vi "Save File.vi"(0 "Save Options":T1={"Component Name"="", "Image Type"=enum."PNG", "Save As"=enum."Save", "Image"=refnum, "PostProcessed?"=FALSE, "Color Palette"=[], "Display Range"={"Maximum"=0, "Minimum"=0}, "Image Refnum"=refnum, "save name"=FALSE, "Dynamic Filter"=FALSE}, 11 "Error in (no error)":errorcluster, 13 "Save Location":enum16{"Primary", "Secondary"}(ring)) -> (4 "Last Saved File Name":string, 8 "Last Saved File Path":path, 15 "Error out":errorcluster)   [LabVIEW 2021]
uses:
  Controls/Save VI States.ctl
  <vilib>/vision/Image Controls.llb/IMAQ Image.ctl
  Controls/Image Type.ctl
  Controls/Save Options.ctl
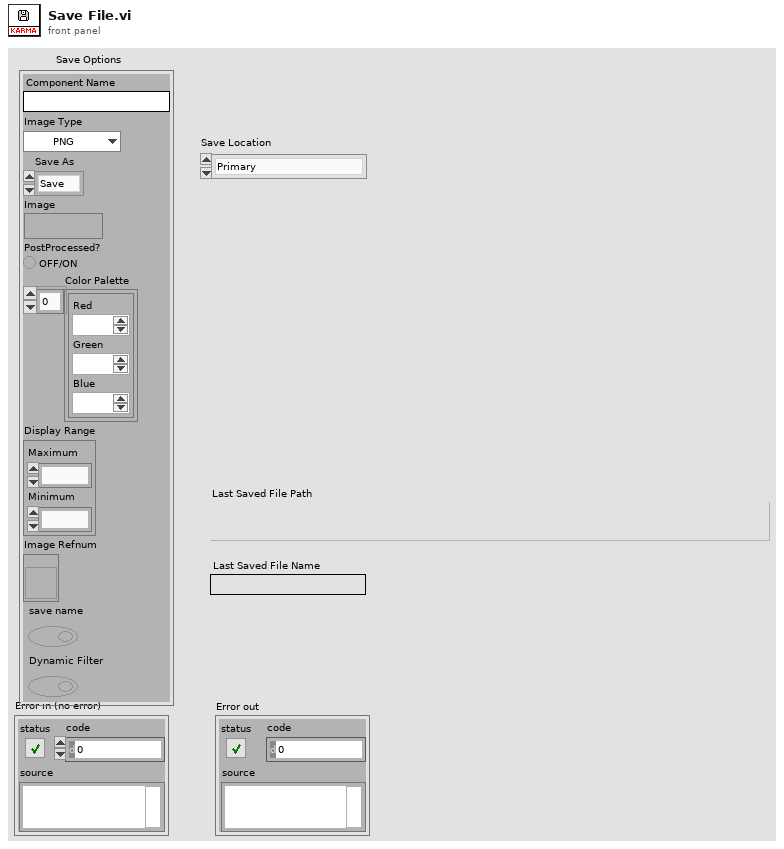
[diagram p1: front panel]
types:
  T1 = typedef "Save Options.ctl" = cluster{"Component Name":string, "Image Type":T2, "Save As":enum16{"Save", "SaveAsOK", "SaveAsNOTOK"}, "Image":T3, "PostProcessed?":bool, "Color Palette":cluster{"Red":u8, "Green":u8, "Blue":u8}[], "Display Range":cluster{"Maximum":i32, "Minimum":i32}, "Image Refnum":refnum<vi>, "save name":bool, "Dynamic Filter":bool}
  T2 = typedef "Image Type.ctl" = enum16{"JPEG", "BMP", "PNG", "TIFF", "DICOM", "RAW"}
  T3 = typedef "IMAQ Image.ctl" = refnum<image>
  T4 = typedef "Save VI States.ctl" = enum16{"Initialize", "Check File Paths", "Target Folder Selection", "Check File Count", "Save File", "Exit"}
  T5 = enum16{"Init Counter", "Read Last Value", "Write Last Value", "Reset Counter", "Increment by 1", "Decrement by 1", "Get Current Count"}
  T6 = cluster{"Last Saved Path":path, "Component name":string}
  T7 = typedef "Application Settings.ctl" = cluster{"Sensor Settings":cluster{"Sensor Type Selection":enum32{"IDS Sensor", "Select Sensor"}, "Select Sensor":T8, "Sensor ID":u32, "Bit Depth":enum16{"<Select>", "8 bits", "16 bits"}}, "Save Options":cluster{"Primary Storage Location":path, "Backup Storage Location":path, "Enable Primary":bool, "Enable Secondary":bool}, "Other Settings":cluster{"Show Image Averaging Option":bool}}
  T8 = typedef "IMAQdx.ctl" = refnum<k21>
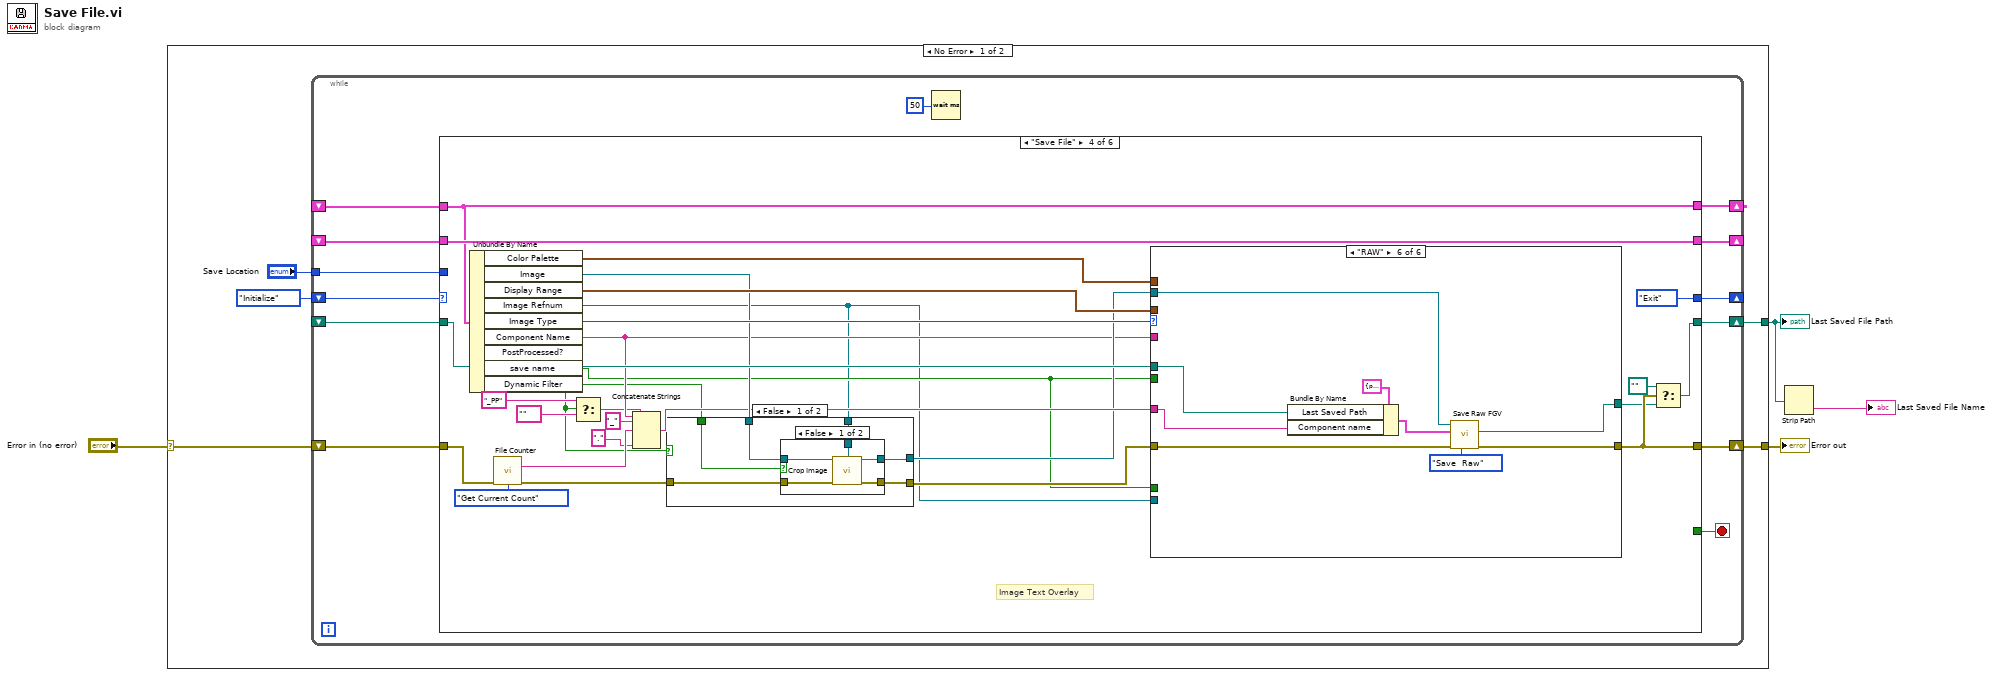
[diagram p0: block diagram]
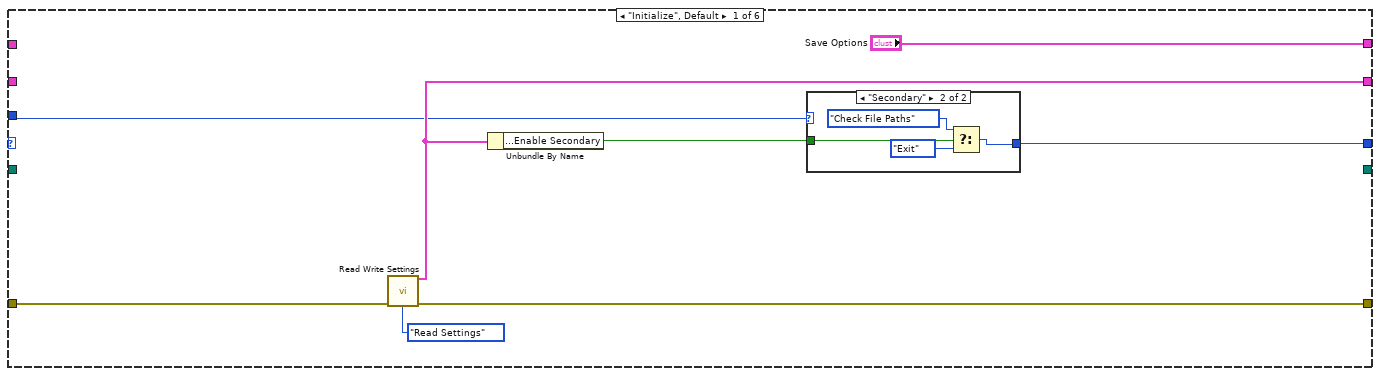
[diagram p2: hidden frame]
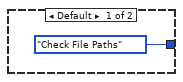
[diagram p3: hidden frame]
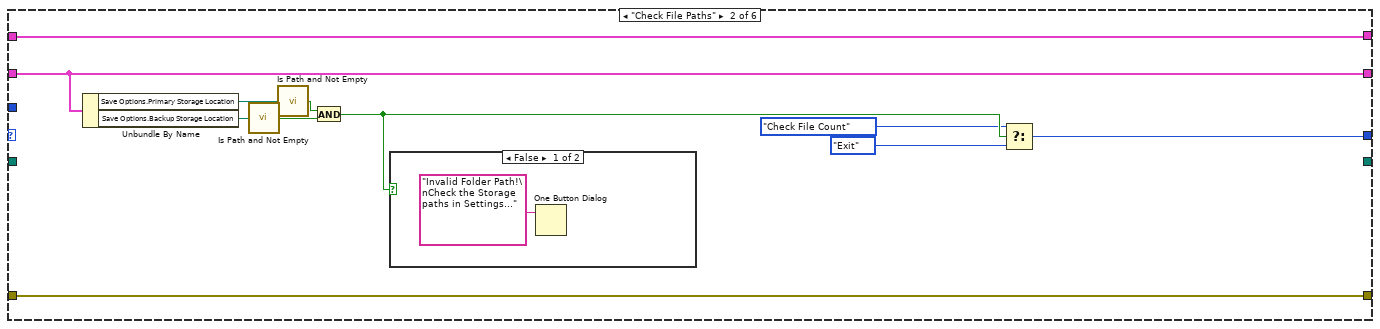
[diagram p4: hidden frame]
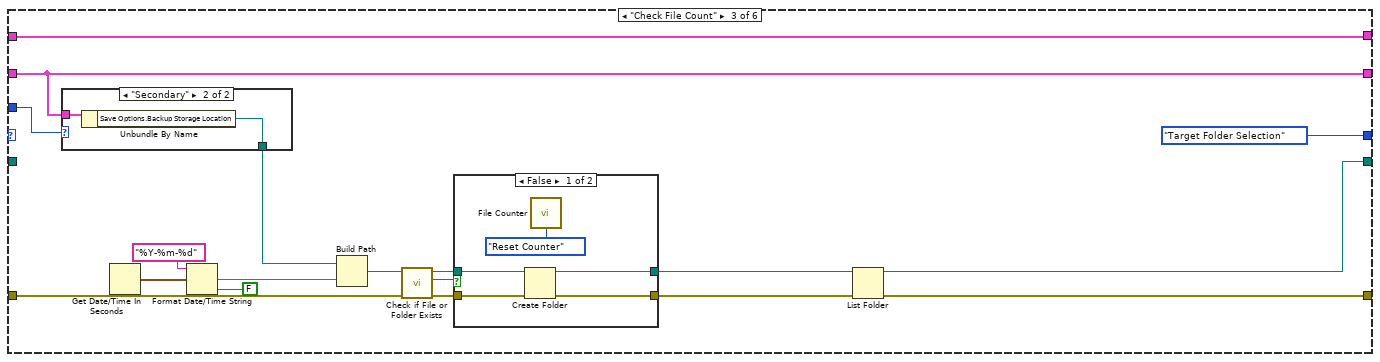
[diagram p6: hidden frame]
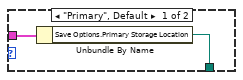
[diagram p7: hidden frame]
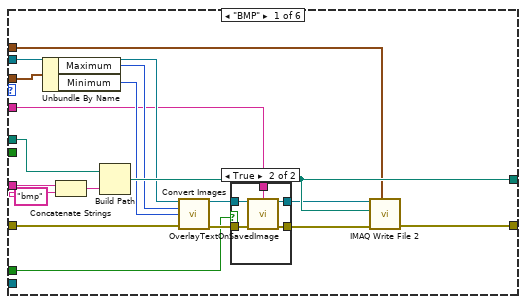
[diagram p11: hidden frame]
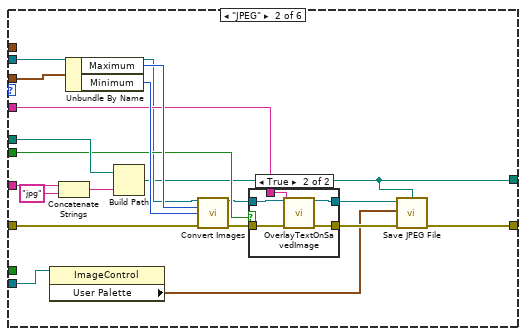
[diagram p13: hidden frame]
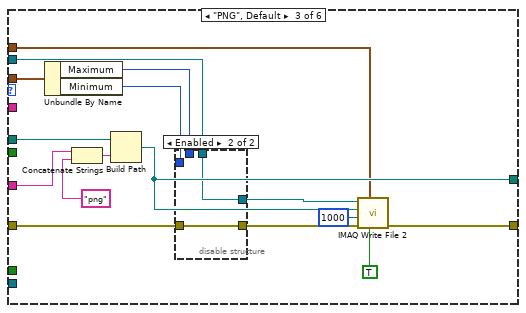
[diagram p15: hidden frame]
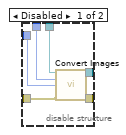
[diagram p16: hidden frame]
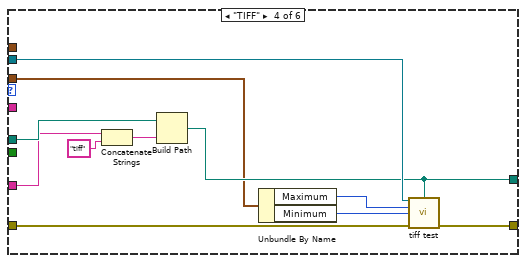
[diagram p17: hidden frame]
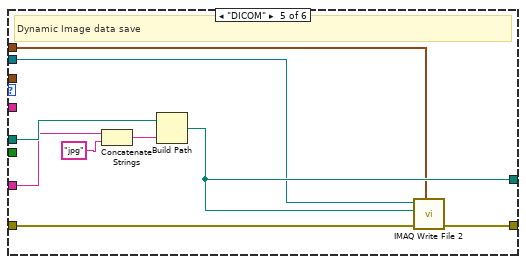
[diagram p18: hidden frame]
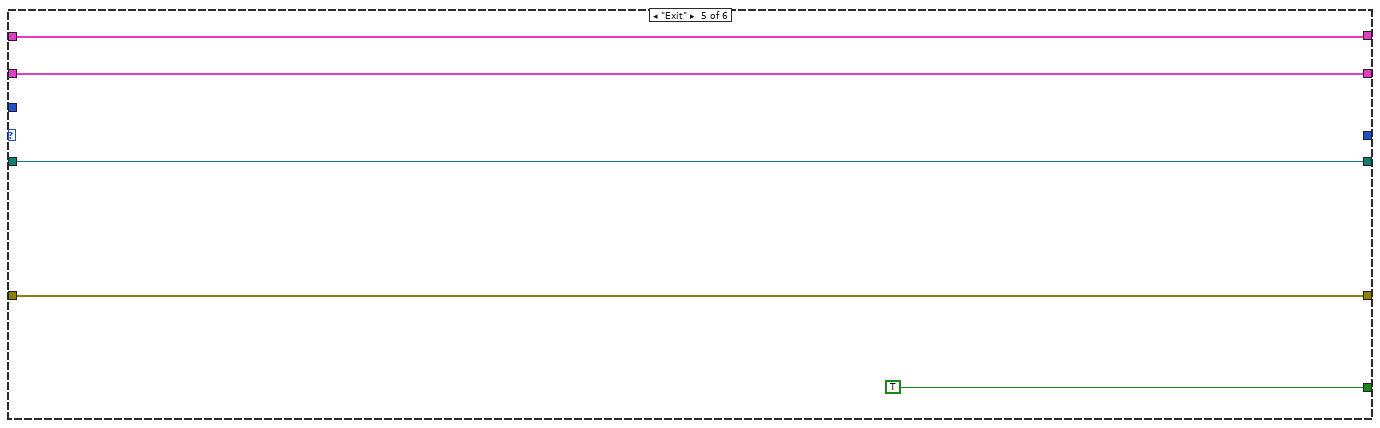
[diagram p19: hidden frame]
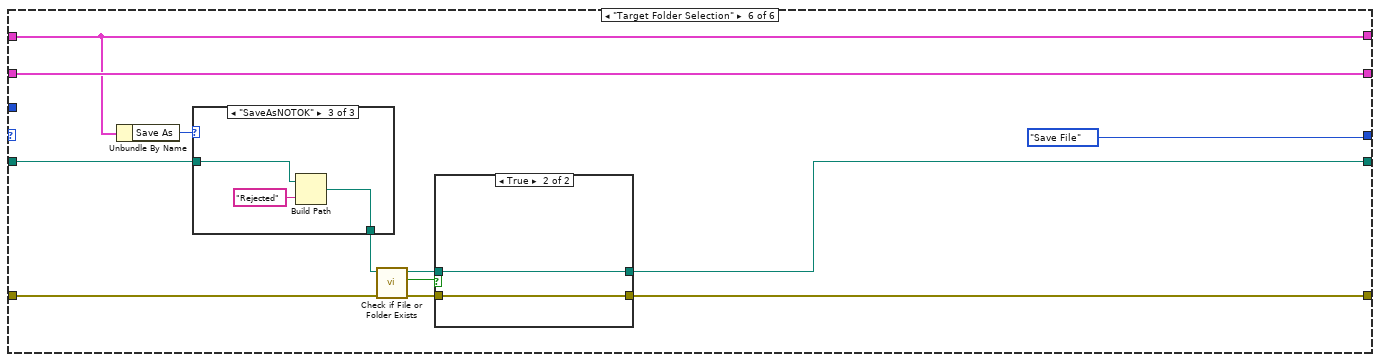
[diagram p20: hidden frame]
diagram:
  n1 = case shown="No Error" "Error in (no error)" {
    selector: "Error in (no error)" -> [w5 w255]
    tunnel: [w7 _] -> w2
    tunnel: [w6 w255] -> w4
    frame No Error {
      n2 = while {
        shift-right: [w14] -> _
        shift-left: Save_VI_States."Initialize" -> [w22]
        shift-right: [w20] -> _
        shift-left: _ -> [w19]
        shift-right: [w16] -> _
        shift-left: _ -> [w15]
        shift-right: [w13] -> w7
        shift-left: _ -> [w12]
        tunnel: "Save Location" -> [w11]
        shift-right: [w17] -> w6
        shift-left: w5 -> [w18]
        stop <- w21 stop-if-true
        n3 = case shown="\"Save File\"" w22 {
          tunnel: [_ _ _ _ TRUE _] -> w21
          tunnel: ["Save Options" w46 w65 w102 w228 w240] -> w20
          tunnel: w19 -> [_ w46 w65 w102 w228 w240]
          tunnel: w18 -> [w28 w38 w53 w89 w226 w233]
          tunnel: [w27 w38 w52 w97 w226 w232] -> w17
          tunnel: [w26 w41 w51 w105 w227 w241] -> w16
          tunnel: w15 -> [_ w41 w51 w105 w227 w241]
          tunnel: [w23 w39 Save_VI_States."Target Folder Selection" Save_VI_States."Exit" _ Save_VI_States."Save File"] -> w14
          tunnel: [_ _ w50 w94 w225 w231] -> w13
          tunnel: w12 -> [_ _ _ w98 w225 w234]
          tunnel: w11 -> [w25 _ w48 _ _ _]
          frame "Initialize", Default {
            n4 = call "Read Write Settings.vi"("error in (no error)"=w28, "Operations"=enum16{"Read Settings", "Write Settings"}."Read Settings") -> ("Settings Out"=w26:T7, "error out"=w27:errorcluster)  [unwired: 12 in]
            n5 = Unbundle By Name(w26) -> ("Save Options.Enable Secondary"=w24:bool)
            n6 = case shown="\"Secondary\"" w25 {
              tunnel: w24 -> [_ w35]
              tunnel: [Save_VI_States."Check File Paths" w33] -> w23
              frame Default {
              }
              frame "Secondary" {
                n7 = Select(t=Save_VI_States."Check File Paths", s=w35, f=Save_VI_States."Exit") -> (s? t:f=w33:T4)
              }
            }
          }
          frame "Check File Paths" {
            n8 = Unbundle By Name(w41) -> ("Save Options.Primary Storage Location"=w43:path, "Save Options.Backup Storage Location"=w42:path)
            n9 = call <vilib>:"Is Path and Not Empty.vi"("path"=w42) -> ("Is Path and Not Empty?"=w45:bool)  [unwired: 4 in]
            n10 = call <vilib>:"Is Path and Not Empty.vi"("path"=w43) -> ("Is Path and Not Empty?"=w44:bool)  [unwired: 4 in]
            n11 = And(x=w44, y=w45) -> (x .and. y?=w40:bool)
            n12 = case shown="False" w40 {
              frame False {
                n13 = One Button Dialog(message="Invalid Folder Path!\nCheck the Storage paths in Settings...") -> ()  [unwired: 1 in, 1 out]
              }
              frame True {
              }
            }
            n14 = Select(t=Save_VI_States."Check File Count", s=w40, f=Save_VI_States."Exit") -> (s? t:f=w39:T4)
          }
          frame "Check File Count" {
            n15 = case shown="\"Secondary\"" w48 {
              tunnel: [w67 w68] -> w54
              tunnel: w51 -> [w66 w69]
              frame "Primary", Default {
                n16 = Unbundle By Name(w66) -> ("Save Options.Primary Storage Location"=w67:path)
              }
              frame "Secondary" {
                n17 = Unbundle By Name(w69) -> ("Save Options.Backup Storage Location"=w68:path)
              }
            }
            n18 = Get Date/Time In Seconds() -> (seconds since 1Jan1904=w58:timestamp)
            n19 = Format Date/Time String(time format string (%c)="%Y-%m-%d", seconds (now)=w58, UTC format=FALSE) -> (date/time string=w55:string)
            n20 = Build Path(base path=w54, name or relative path=w55) -> (appended path=w64:path)
            n21 = call <vilib>:"Check if File or Folder Exists.vi"("error in (no error)"=w53, "path"=w64) -> ("error out"=w62:errorcluster, "file or folder exists?"=w63:bool, "dup path"=w61:path)  [unwired: 7 in]
            n22 = case shown="False" w63 {
              tunnel: w62 -> [w74 w76]
              tunnel: w61 -> [w72 w75]
              tunnel: [w73 w76] -> w60
              tunnel: [w71 w75] -> w59
              frame False {
                n23 = Create Folder(path (use dialog)=w72, error in=w74) -> (created path=w71:path, error out=w73:errorcluster)  [unwired: 1 in, 1 out]
                n24 = call "File Counter.vi"("Operations"=T5."Reset Counter") -> ()  [unwired: 12 in, 3 out]
              }
              frame True {
              }
            }
            n25 = List Folder(path=w59, error in=w60) -> (path out=w50:path, error out=w52:errorcluster)  [unwired: 2 in, 2 out]
          }
          frame "Save File" {
            # "Image Text Overlay"
            n26 = Unbundle By Name(w102) -> ("Color Palette"=w90:cluster{"Red":u8, "Green":u8, "Blue":u8}[], "Image"=w86:T3, "Display Range"=w91:cluster{"Maximum":i32, "Minimum":i32}, "Image Refnum"=w80:refnum<vi>, "Image Type"=w99:T2, "Component Name"=w82:string, "PostProcessed?"=w87:bool, "save name"=w81:bool, "Dynamic Filter"=w79:bool)
            n27 = call "File Counter.vi"("Error in"=w89, "Operations"=T5."Get Current Count") -> ("Count"=w100:string, "Error out"=w88:errorcluster)  [unwired: 11 in, 1 out]
            n28 = Select(t="_PP" ("string"), s=w87, f="") -> (s? t:f=w77:string)
            n29 = Concatenate Strings(w82, "_" ("f"), w100, w77, "." ("string")) -> (w85:string)
            n30 = case shown="False" w87 {
              tunnel: [w110 w119] -> w84
              tunnel: w86 -> [w109 w120]
              tunnel: [w108 w120] -> w83
              tunnel: w88 -> [w111 w119]
              tunnel: w80 -> [w107 _]
              tunnel: w79 -> [w106 _]
              frame False {
                n31 = case shown="False" w106 {
                  tunnel: w111 -> [w116 w117]
                  tunnel: [w115 w117] -> w110
                  tunnel: w109 -> [w114 w118]
                  tunnel: [w113 w118] -> w108
                  tunnel: w107 -> [w112 _]
                  frame False {
                    n32 = call "Crop Image.vi"("Image Src"=w114, "Image Refnum"=w112, "Error in (no error)"=w116) -> ("Cropped Image"=w113:T3, "Error in (no error)"=w115:errorcluster)  [unwired: 11 in]
                  }
                  frame True {
                  }
                }
              }
              frame True {
              }
            }
            n33 = case shown="\"RAW\"" w99 {
              tunnel: w84 -> [w132 w154 w177 w202 w215 w224]
              tunnel: [w138 w150 w187 w201 w214 w223] -> w97
              tunnel: w85 -> [w134 w163 w186 w203 w210 w216]
              tunnel: w98 -> [w135 w164 w185 w204 w211 w221]
              tunnel: [w133 w149 w182 w199 w209 w217] -> w96
              tunnel: w83 -> [w131 w155 w175 w200 w208 w220]
              tunnel: w91 -> [w129 w160 w178 w198 _ _]
              tunnel: w90 -> [w130 _ w179 _ w207 _]
              tunnel: w82 -> [w122 w157 _ _ _ _]
              tunnel: w81 -> [w121 _ _ _ _ _]
              tunnel: w81 -> [_ w156 _ _ _ _]
              tunnel: w80 -> [_ w147 _ _ _ _]
              frame "BMP" {
                n34 = Unbundle By Name(w129) -> ("Maximum"=w128:i32, "Minimum"=w127:i32)
                n35 = Concatenate Strings(w134, "bmp" ("string")) -> (w137:string)
                n36 = Build Path(base path=w135, name or relative path=w137) -> (appended path=w133:path)
                n37 = call "Convert Images.vi"("Image In"=w131, "Max Value"=w128, "Min Value"=w127, "Error in (no error)"=w132) -> ("Image Out"=w124:T3, "Error out"=w126:errorcluster)  [unwired: 10 in]
                n38 = case shown="True" w121 {
                  tunnel: w126 -> [w139 w145]
                  tunnel: [w139 w144] -> w125
                  tunnel: w124 -> [w140 w143]
                  tunnel: [w140 w142] -> w123
                  tunnel: w122 -> [_ w141]
                  frame False {
                  }
                  frame True {
                    n39 = call "OverlayTextOnSavedImage.vi"("Image"=w143, "Component Name"=w141, "Error in (no error)"=w145) -> ("Image Dst Out"=w142:T3, "Error out"=w144:errorcluster)  [unwired: 11 in]
                  }
                }
                n40 = call-poly "IMAQ Write File 2"("Color Palette"=w130, "error in (no error)"=w125, "File Path"=w133, "Image"=w123) -> ("error out"=w138:errorcluster)  [unwired: 6 in, 1 out]
              }
              frame "JPEG" {
                n41 = property class="ImageControl"(reference=w147) -> ("User Palette"=w146:cluster{"Red":u8, "Green":u8, "Blue":u8}[])  [unwired: 1 in, 2 out]
                n42 = Concatenate Strings(w163, "jpg" ("string")) -> (w161:string)
                n43 = Unbundle By Name(w160) -> ("Maximum"=w159:i32, "Minimum"=w158:i32)
                n44 = Build Path(base path=w164, name or relative path=w161) -> (appended path=w149:path)
                n45 = call "Convert Images.vi"("Image In"=w155, "Max Value"=w159, "Min Value"=w158, "Error in (no error)"=w154) -> ("Image Out"=w152:T3, "Error out"=w153:errorcluster)  [unwired: 10 in]
                n46 = case shown="True" w156 {
                  tunnel: w152 -> [w166 w171]
                  tunnel: [w166 w170] -> w148
                  tunnel: w153 -> [w165 w169]
                  tunnel: [w165 w168] -> w151
                  tunnel: w157 -> [_ w167]
                  frame False {
                  }
                  frame True {
                    n47 = call "OverlayTextOnSavedImage.vi"("Image"=w171, "Component Name"=w167, "Error in (no error)"=w169) -> ("Image Dst Out"=w170:T3, "Error out"=w168:errorcluster)  [unwired: 11 in]
                  }
                }
                n48 = call "Save JPEG File.vi"("Image In"=w148, "Color Palette In"=w146, "Error in (no error)"=w151, "JPEG File Path"=w149) -> ("Error out"=w150:errorcluster)  [unwired: 10 in, 1 out]
              }
              frame "PNG", Default {
                n49 = Unbundle By Name(w178) -> ("Maximum"=w173:i32, "Minimum"=w172:i32)
                n50 = Concatenate Strings(w186, "png" ("string")) -> (w184:string)
                n51 = Build Path(base path=w185, name or relative path=w184) -> (appended path=w182:path)
                n52 = disable-structure shown="Enabled" {
                  disable-tunnel: w177 -> [w193 w195]
                  disable-tunnel: [w192 w195] -> w176
                  disable-tunnel: w175 -> [w191 w194]
                  disable-tunnel: [w190 w194] -> w174
                  disable-tunnel: w173 -> [w189 _]
                  disable-tunnel: w172 -> [w188 _]
                  frame Disabled {
                    n53 = call "Convert Images.vi"("Image In"=w191, "Max Value"=w189, "Min Value"=w188, "Error in (no error)"=w193) -> ("Image Out"=w190:T3, "Error out"=w192:errorcluster)  [unwired: 10 in]
                  }
                  frame Enabled {
                  }
                }
                n54 = call-poly "IMAQ Write File 2"("Use bit depth? (false)"=TRUE, "Color Palette"=w179, "error in (no error)"=w176, "Image Quality"=u32 1000, "File Path"=w182, "Image"=w174) -> ("error out"=w187:errorcluster)  [unwired: 4 in, 1 out]
              }
              frame "TIFF" {
                n55 = Concatenate Strings(w203, "tiff" ("string")) -> (w206:string)
                n56 = Build Path(base path=w204, name or relative path=w206) -> (appended path=w199:path)
                n57 = Unbundle By Name(w198) -> ("Maximum"=w197:i32, "Minimum"=w196:i32)
                n58 = call "tiff test.vi"("Image In"=w200, "Target File Path"=w199, "Max"=w197, "Min"=w196, "Error in (no error)"=w202) -> ("Error out"=w201:errorcluster)  [unwired: 9 in, 1 out]
              }
              frame "DICOM" {
                # "Dynamic Image data save"
                n59 = Concatenate Strings(w210, "jpg" ("string")) -> (w213:string)
                n60 = Build Path(base path=w211, name or relative path=w213) -> (appended path=w209:path)
                n61 = call-poly "IMAQ Write File 2"("Color Palette"=w207, "error in (no error)"=w215, "File Path"=w209, "Image"=w208) -> ("error out"=w214:errorcluster)  [unwired: 6 in, 1 out]
              }
              frame "RAW" {
                n62 = Bundle By Name(cluster=T6 {"Last Saved Path"=path "", "Component name"=""} ("Data Cluster"), "Last Saved Path"=w221, "Component name"=w216) -> (w218:T6)
                n63 = call "Save Raw FGV.vi"("Save Options"=enum16{"Save  Raw", "Fetch Raw", "Error"}."Save  Raw", "error in (no error)"=w224, "Data Cluster"=w218, "Image In"=w220) -> ("error out"=w223:errorcluster, "File Name"=w217:path)  [unwired: 5 in, 1 out]
              }
            }
            n64 = Select(t=path "", s=w97, f=w96) -> (s? t:f=w94:path)
          }
          frame "Exit" {
          }
          frame "Target Folder Selection" {
            n65 = Unbundle By Name(w240) -> ("Save As"=w235:enum16{"Save", "SaveAsOK", "SaveAsNOTOK"})
            n66 = case shown="\"SaveAsNOTOK\"" w235 {
              tunnel: [w242 w245 w246] -> w239
              tunnel: w234 -> [w242 w244 w247]
              frame "Save", Default {
              }
              frame "SaveAsOK" {
                n67 = Build Path(base path=w244, name or relative path="Accepted") -> (appended path=w245:path)
              }
              frame "SaveAsNOTOK" {
                n68 = Build Path(base path=w247, name or relative path="Rejected") -> (appended path=w246:path)
              }
            }
            n69 = call <vilib>:"Check if File or Folder Exists.vi"("error in (no error)"=w233, "path"=w239) -> ("error out"=w237:errorcluster, "file or folder exists?"=w238:bool, "dup path"=w236:path)  [unwired: 7 in]
            n70 = case shown="True" w238 {
              tunnel: w237 -> [w252 w254]
              tunnel: w236 -> [w250 w253]
              tunnel: [w251 w254] -> w232
              tunnel: [w249 w253] -> w231
              frame False {
                n71 = Create Folder(path (use dialog)=w250, error in=w252) -> (created path=w249:path, error out=w251:errorcluster)  [unwired: 1 in, 1 out]
              }
              frame True {
              }
            }
          }
        }
        n72 = Wait (ms)(milliseconds to wait=u32 50) -> ()  [unwired: 1 out]
      }
    }
    frame Error {
    }
  }
  "Error out" <- w4
  "Last Saved File Path" <- w2
  n73 = Strip Path(path=w2) -> (name=→"Last Saved File Name":string)  [unwired: 1 out]
